vi "velosterpaserraw.vi"(0 "roll":dbl=0.5000000000000001, 1 "pitch":dbl=-6.0, 2 "heading":dbl=1.2, 3 "dX":dbl=-0.009999999999999997, 4 "dY":dbl=1.287, 5 "dZ":dbl=1.6) -> ()   [LabVIEW 2015]
uses:
  G_SEN.vi
  <vilib>/Analysis/Matrix/Numeric/Conversions/Array To Matrix - RA2.vi
  <vilib>/Analysis/Matrix/Numeric/Multiply/Multiply - RM,RM.vi
  <vilib>/Analysis/Matrix/NI_Matrix.lvlib
panel:
  in  "Velodyne":T1(ring)=enum."Velodyne 64"
  out "XY Graph 2":cluster{"X":dbl, "Y":dbl}[](graph)
  out "X":dbl[](array[numeric])
  out "Y":dbl[](array[numeric])
  out "Z":dbl[](array[numeric])
  out "d":dbl[](array[numeric])
  out "i":u8[](array[numeric])
  in  "thresh":dbl
  out "pos_velo":dbl[](array[numeric])
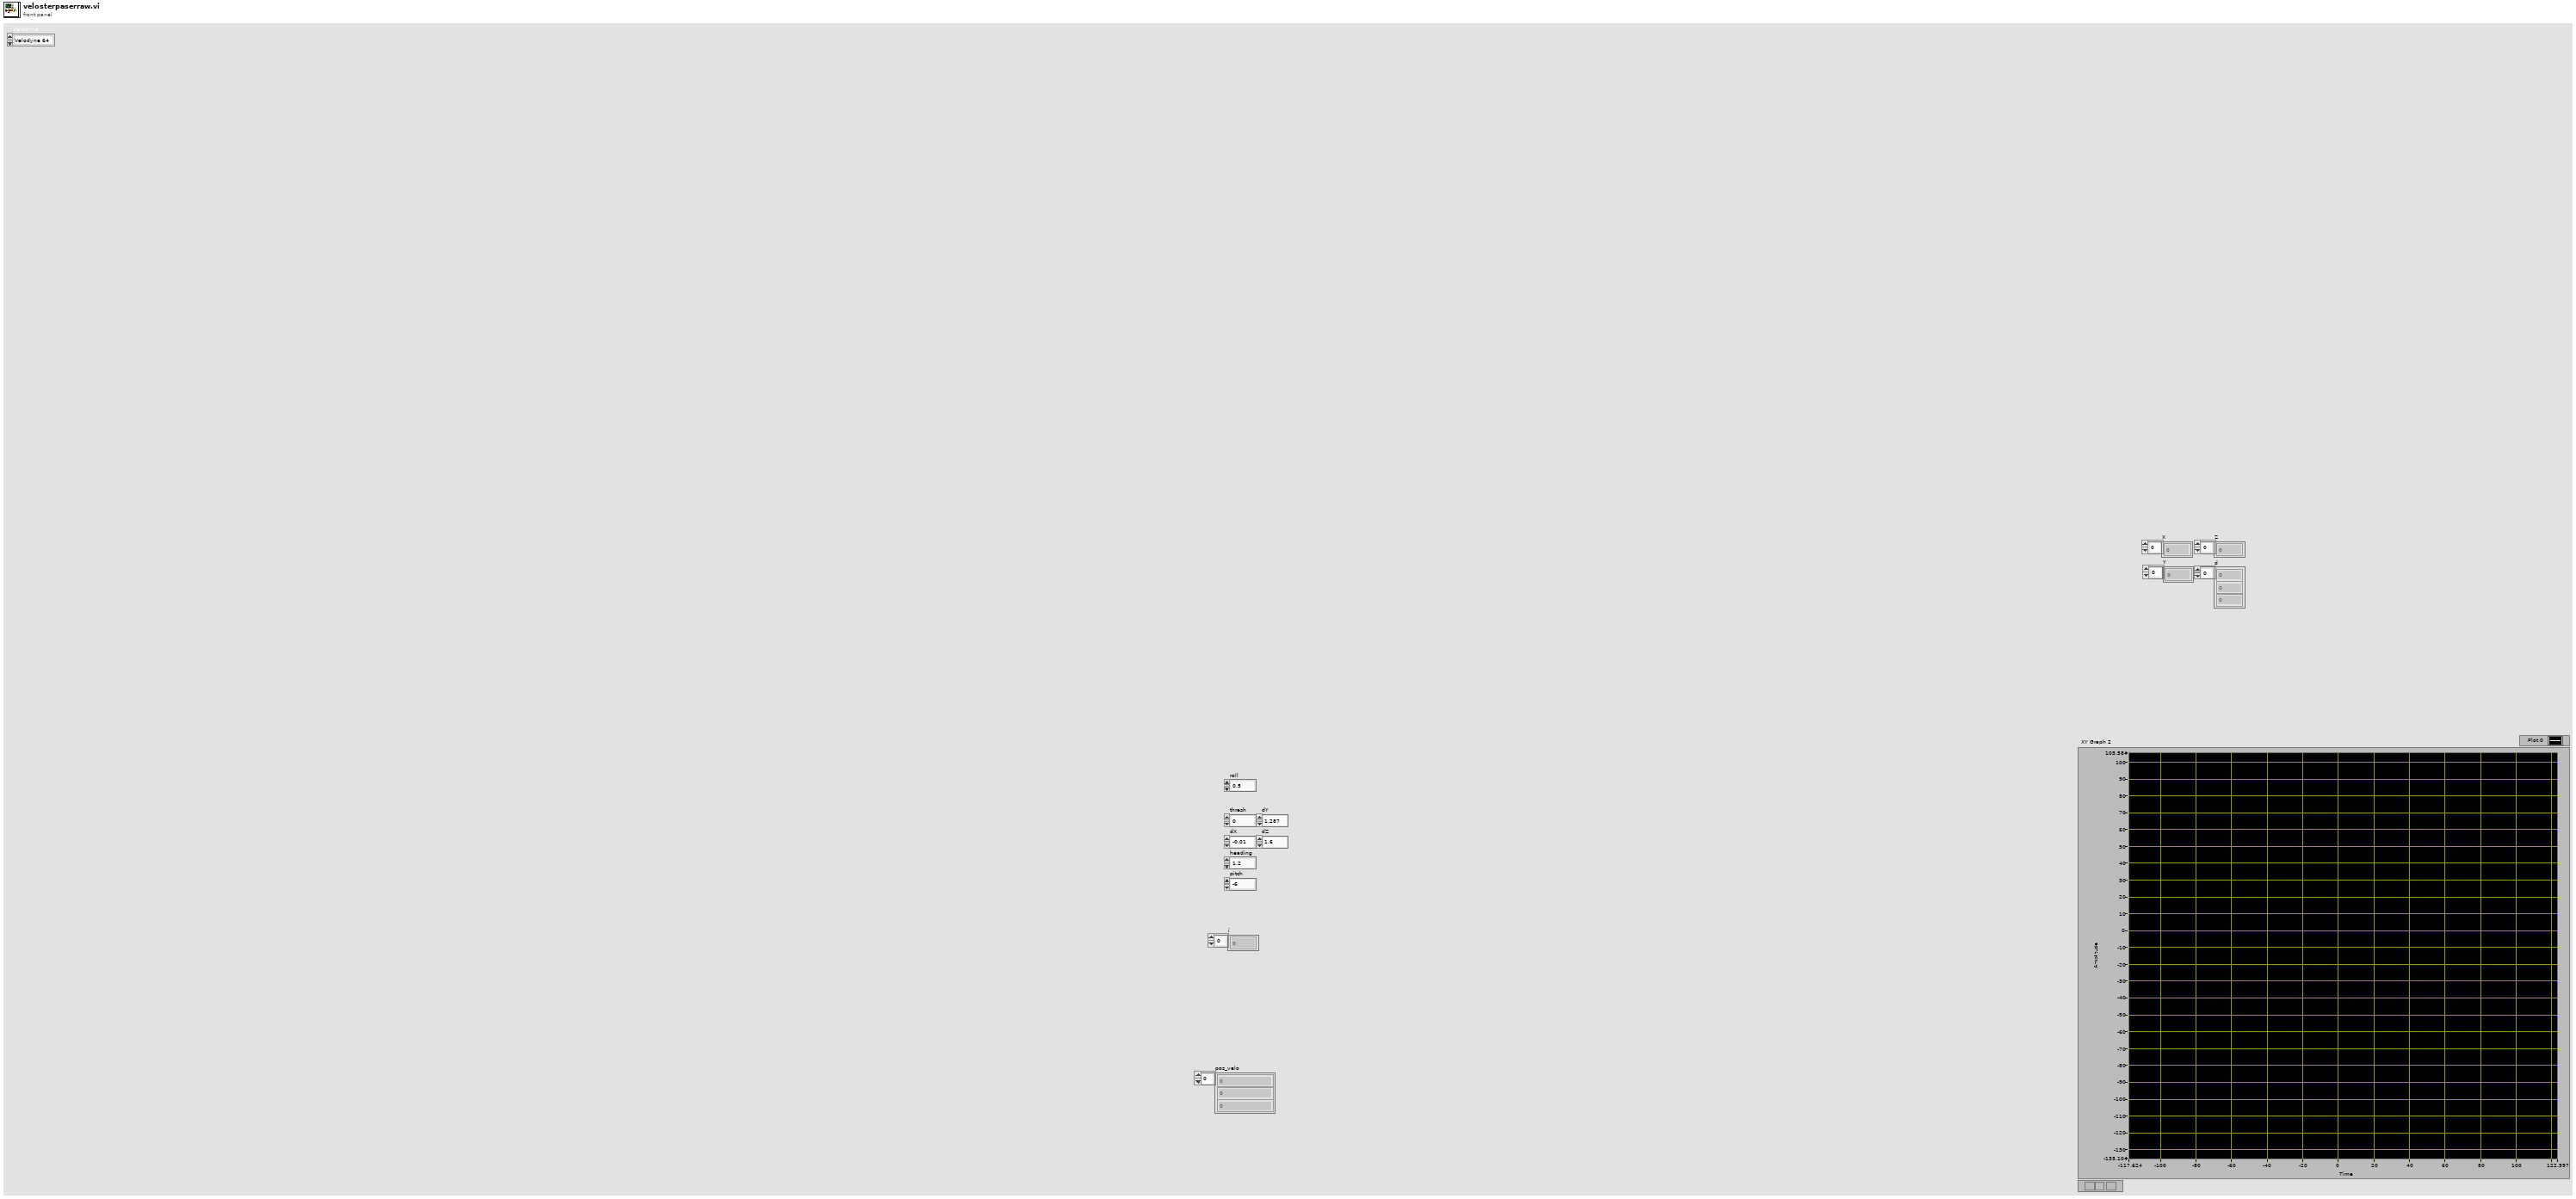
[diagram p1: front panel]
types:
  T1 = enum16{"Velodyne 16", "Velodyne 32", "Velodyne 64"}
  T2 = cluster{"X":dbl[], "Y":dbl[], "Z":dbl[], "d":dbl[], "i":u8[]}
  T3 = typedef "NI_Matrix.lvlib/RealMatrix.ctl" = dbl[][]
  T4 = cluster{i16, dbl, dbl, dbl, "Rotational position":dbl, "element":u8}[]
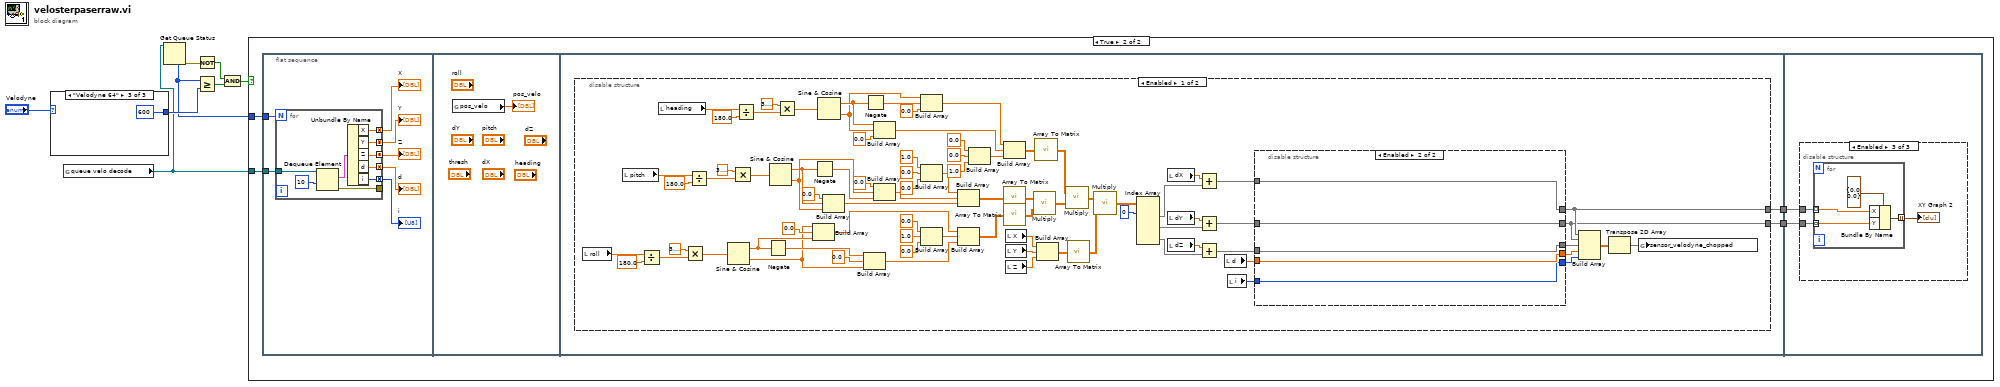
[diagram p0: block diagram]
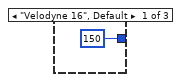
[diagram p2: hidden frame]
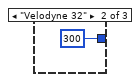
[diagram p3: hidden frame]
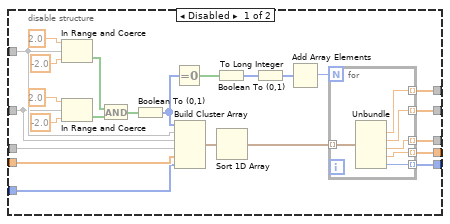
[diagram p5: hidden frame]
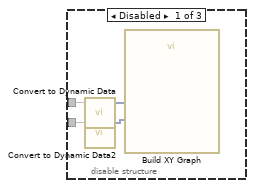
[diagram p7: hidden frame]
diagram:
  n1 = case shown="\"Velodyne 64\"" "Velodyne" {
    tunnel: [150 300 600] -> w5
    frame "Velodyne 16", Default {
    }
    frame "Velodyne 32" {
    }
    frame "Velodyne 64" {
    }
  }
  n2 = global read "G_SEN.vi" "queue velo decode"() -> (w1:refnum<queue>)
  n3 = Get Queue Status(queue=w1) -> (error out=w7:errorcluster, # elements in queue=w3:i32)  [unwired: 2 in, 6 out]
  n4 = Not(x=w7) -> (.not. x?=w6:bool)
  n5 = Greater Or Equal?(x=w3, y=w5) -> (x >= y?=w8:bool)
  n6 = And(x=w6, y=w8) -> (x .and. y?=w4:bool)
  n7 = case shown="True" w4 {
    tunnel: w3 -> [_ w12]
    tunnel: w1 -> [_ w13]
    frame False {
    }
    frame True {
      n8 = flat-sequence {
        tunnel: w13 -> [w22]
        tunnel: w12 -> [w21]
        tunnel: [w34] -> w15
        tunnel: [w33] -> w14
        tunnel: w15 -> [w152]
        tunnel: w14 -> [w151]
        frame #0 {
          n9 = for {
            N: w21 -> [_]
            tunnel: w22 -> [w31]
            tunnel: [w29] -> w20 mode=concatenating
            tunnel: [w28] -> w19 mode=concatenating
            tunnel: [w27] -> w18 mode=concatenating
            tunnel: [w26] -> w17 mode=concatenating
            tunnel: [w25] -> w16 mode=concatenating
            tunnel: [w24] -> _
            n10 = Dequeue Element(queue=w31, timeout in ms (-1)=10) -> (element=w30:T2, error out=w24:errorcluster)  [unwired: 1 in, 2 out]
            n11 = Unbundle By Name(w30) -> ("X"=w29:dbl[], "Y"=w28:dbl[], "Z"=w27:dbl[], "d"=w26:dbl[], "i"=w25:u8[])
          }
          "X" <- w20
          "Y" <- w19
          "Z" <- w18
          "d" <- w17
          "i" <- w16
        }
        frame #1 {
          n12 = global read "G_SEN.vi" "pos_velo"() -> (→"pos_velo":dbl[])
        }
        frame #2 {
          n13 = disable-structure shown="Enabled" {
            disable-tunnel: [w36 _] -> w34
            disable-tunnel: [w35 _] -> w33
            frame Enabled {
              n14 = local read "roll"() -> (w48:dbl)
              n15 = local read "pitch"() -> (w57:dbl)
              n16 = Divide(x=w48, y=180.0) -> (x/y=w50:dbl)
              n17 = local read "heading"() -> (w52:dbl)
              n18 = Multiply(x=3.141592653589793, y=w50) -> (x*y=w46:dbl)
              n19 = Divide(x=w57, y=180.0) -> (x/y=w60:dbl)
              n20 = Sine & Cosine(0:w46) -> (1:w102:dbl, 2:w99:dbl)
              n21 = Multiply(x=3.141592653589793, y=w60) -> (x*y=w56:dbl)
              n22 = Divide(x=w52, y=180.0) -> (x/y=w53:dbl)
              n23 = Negate(x=w102) -> (-x=w101:dbl)
              n24 = Sine & Cosine(0:w56) -> (1:w86:dbl, 2:w89:dbl)
              n25 = Multiply(x=3.141592653589793, y=w53) -> (x*y=w51:dbl)
              n26 = Build Array(w99, 0.0 ("element"), w102) -> (w104:dbl[])
              n27 = Negate(x=w86) -> (-x=w88:dbl)
              n28 = Sine & Cosine(0:w51) -> (1:w83:dbl, 2:w81:dbl)
              n29 = Build Array(0.0 ("element"), w86, w89) -> (w85:dbl[])
              n30 = Build Array(w101, 0.0 ("element"), w99) -> (w98:dbl[])
              n31 = Negate(x=w83) -> (-x=w82:dbl)
              n32 = Build Array(w83, w81, 0.0 ("element")) -> (w84:dbl[])
              n33 = Build Array(0.0 ("element"), w89, w88) -> (w91:dbl[])
              n34 = Build Array(w81, w82, 0.0 ("element")) -> (w80:dbl[])
              n35 = Build Array(1.0 ("element"), 0.0 ("element"), 0.0 ("element")) -> (w92:dbl[])
              n36 = Build Array(0.0 ("element"), 1.0 ("element"), 0.0 ("element")) -> (w103:dbl[])
              n37 = Build Array(w92, w91, w85) -> (w96:dbl[][])
              n38 = Build Array(w104, w103, w98) -> (w97:dbl[][])
              n39 = Build Array(0.0 ("element"), 0.0 ("element"), 1.0 ("element")) -> (w75:dbl[])
              n40 = Build Array(w80, w84, w75) -> (w76:dbl[][])
              n41 = call-poly <vilib>:"Array To Matrix.vi"("Real 2D Array"=w96) -> ("Real Matrix"=w71:T3)
              n42 = call-poly <vilib>:"Array To Matrix.vi"("Real 2D Array"=w97) -> ("Real Matrix"=w72:T3)
              n43 = local read "X"() -> (w68:dbl[])
              n44 = local read "Y"() -> (w67:dbl[])
              n45 = local read "Z"() -> (w66:dbl[])
              n46 = call-poly <vilib>:"Multiply.vi"("Real Matrix B"=w72, "Real Matrix A"=w71) -> ("A * B"=w70:T3)
              n47 = call-poly <vilib>:"Array To Matrix.vi"("Real 2D Array"=w76) -> ("Real Matrix"=w69:T3)
              n48 = Build Array(w68, w67, w66) -> (w65:dbl[][])
              n49 = call-poly <vilib>:"Multiply.vi"("Real Matrix B"=w70, "Real Matrix A"=w69) -> ("A * B"=w64:T3)
              n50 = call-poly <vilib>:"Array To Matrix.vi"("Real 2D Array"=w65) -> ("Real Matrix"=w63:T3)
              n51 = call-poly <vilib>:"Multiply.vi"("Real Matrix B"=w63, "Real Matrix A"=w64) -> ("A * B"=w62:T3)
              n52 = Index Array(array=w62, index (row) #1=0 ("index (row)")) -> (element #1=w111:dbl[], element #2=w113:dbl[], element #3=w115:dbl[])  [unwired: 5 in]
              n53 = local read "dX"() -> (w110:dbl)
              n54 = local read "dY"() -> (w112:dbl)
              n55 = local read "dZ"() -> (w114:dbl)
              n56 = Add(x=w110, y=w111) -> (x+y=w44:dbl[])
              n57 = Add(x=w112, y=w113) -> (x+y=w41:dbl[])
              n58 = Add(x=w114, y=w115) -> (x+y=w109:dbl[])
              n59 = local read "d"() -> (w43:dbl[])
              n60 = local read "i"() -> (w42:u8[])
              n61 = disable-structure shown="Enabled" {
                disable-tunnel: w109 -> [w139 w148]
                disable-tunnel: w44 -> [w131 w150]
                disable-tunnel: w43 -> [w130 w147]
                disable-tunnel: w42 -> [w129 w146]
                disable-tunnel: [w123 w150] -> w36
                disable-tunnel: w41 -> [w122 w149]
                disable-tunnel: [w121 w149] -> w35
                disable-tunnel: [w120 w148] -> w40
                disable-tunnel: [w119 w147] -> w39
                disable-tunnel: [w118 w146] -> w38
                frame Disabled {
                  n62 = In Range and Coerce(upper limit=2.0, x=w131, lower limit=-2.0) -> (In Range?=w136:bool[])  [unwired: 1 out]
                  n63 = In Range and Coerce(upper limit=2.0, x=w122, lower limit=-2.0) -> (In Range?=w133:bool[])  [unwired: 1 out]
                  n64 = And(x=w136, y=w133) -> (x .and. y?=w132:bool[])
                  n65 = Boolean To (0,1)(Boolean=w132) -> (0, 1=w127:i16[])
                  n66 = Equal To 0?(x=w127) -> (x = 0?=w126:bool[])
                  n67 = Build Cluster Array(w127, w131, w122, w139, w130, w129) -> (w128:T4)
                  n68 = Boolean To (0,1)(Boolean=w126) -> (0, 1=w117:i16[])
                  n69 = Sort 1D Array(array=w128) -> (sorted array=w124:T4)
                  n70 = To Long Integer(number=w117) -> (32bit integer=w116:i32[])
                  n71 = Add Array Elements(numeric array=w116) -> (sum=w125:i32)
                  n72 = for {
                    N: w125 -> [_]
                    tunnel: w124 -> [w145] mode=indexing
                    tunnel: [w144] -> w123 mode=indexing
                    tunnel: [w143] -> w121 mode=indexing
                    tunnel: [w142] -> w120 mode=indexing
                    tunnel: [w141] -> w119 mode=indexing
                    tunnel: [w140] -> w118 mode=indexing
                    n73 = Unbundle(w145) -> (w144:dbl, w143:dbl, w142:dbl, "Rotational position"=w141:dbl, "element"=w140:u8)  [unwired: 1 out]
                  }
                }
                frame Enabled {
                }
              }
              n74 = Build Array(w36, w35, w40, w39, w38) -> (w45:dbl[][])
              n75 = Transpose 2D Array(2D array=w45) -> (transposed array=w37:dbl[][])
              n76 = global write "G_SEN.vi" "sensor_velodyne_chopped"(w37) -> ()
            }
            frame Disabled {
            }
          }
        }
        frame #3 {
          n77 = disable-structure shown="Enabled" {
            disable-tunnel: w152 -> [w154 _ w159]
            disable-tunnel: w151 -> [w153 _ w158]
            frame Disabled {
              n78 = call "Convert to Dynamic Data"("Array"=w154) -> ("Dynamic Data Type"=w156:dynamicdata)  [unwired: 3 in]
              n79 = call "Convert to Dynamic Data2"("Array"=w153) -> ("Dynamic Data Type"=w155:dynamicdata)  [unwired: 3 in]
              n80 = call "Build XY Graph"("Y Input"=w155, "X Input"=w156) -> ("XY Graph"=w157:cluster{"X":dbl[], "Y":dbl[]}[])  [unwired: 8 in, 1 out]
            }
            frame Disabled {
            }
            frame Enabled {
              n81 = for {
                tunnel: w159 -> [w163] mode=indexing
                tunnel: w158 -> [w162] mode=indexing
                tunnel: [w161] -> w160 mode=indexing
                n82 = Bundle By Name(cluster=cluster{"X":dbl, "Y":dbl} {"X"=0.0, "Y"=0.0}, "X"=w163, "Y"=w162) -> (w161:cluster{"X":dbl, "Y":dbl})
              }
              "XY Graph 2" <- w160
            }
          }
        }
      }
    }
  }
